vi "EVS Main Temp.vi"() -> ()   [LabVIEW 2009]
uses:
  <vilib>/vision/driver/NI_Vision_Acquisition_Software.lvlib
  <vilib>/vision/driver/IMAQdx.llb/IMAQdx Acquisition Mode.ctl
  TypeDefs/cRIO-EVS Comm/EVS to cRIO UDP packet.ctl
  UDP Lib/UDP Network Location.ctl
  <vilib>/userDefined/High Color/IMAQdx.ctl
panel:
  out "Peak":u32
  out "Processing time":u32
  in  "stop":bool
  out "Camera SICK":picture
  out "HB":bool
  in  "IMAQdx Session Left":T1="cam1" caption="Left Session"
  in  "IMAQdx Session Right":T1="cam0" caption="Right Session"
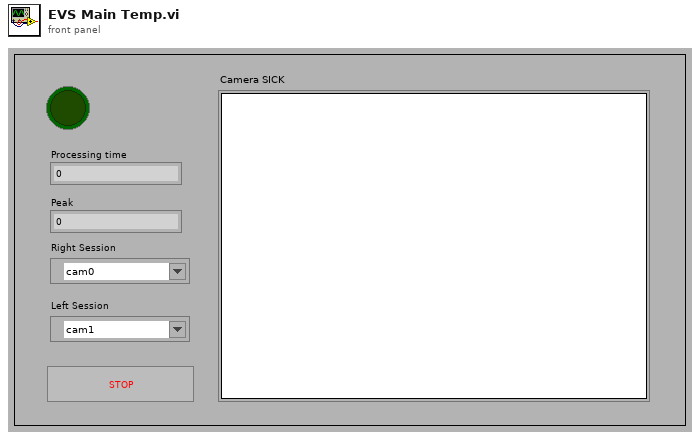
[diagram p1: front panel]
types:
  T1 = typedef "IMAQdx.ctl" = refnum<k21>
  T2 = typedef "UDP Network Location.ctl" = cluster{"IP Address":string, "Port":u16}
  T3 = typedef "EVS to cRIO UDP packet.ctl" = cluster{"Camera SICK":u16[], "Camera init":bool}
  T4 = typedef "NI_Vision_Acquisition_Software.lvlib/IMAQdx Acquisition Mode.ctl" = enum32{"One Shot", "Continuous"}
  T5 = cluster{"maximum":dbl, "minimum":dbl, "clip to min":bool, "log?(F)":bool, "grid color":u32, "plot color":u32, "fmt and prec":cluster{"format":enum8{"Decimal", "Scientific", "Engineering", "Binary", "Octal", "Hex"}, "precision":u8}, "visible section":u16}
  T6 = typedef "UDP Base.ctl" = cluster{"UDP Session":refnum<k16>, "UDP Socket Params":T7}
  T7 = typedef "UDP Socket Params.ctl" = cluster{"Local Port":u16, "Read Timeout":i32, "Write Timeout":i32}
  T8 = typedef "IMAQ Image.ctl" = refnum<image>
  T9 = cluster{"Camera SICK":u16[], ".not. x?":bool, "error out":errorcluster}
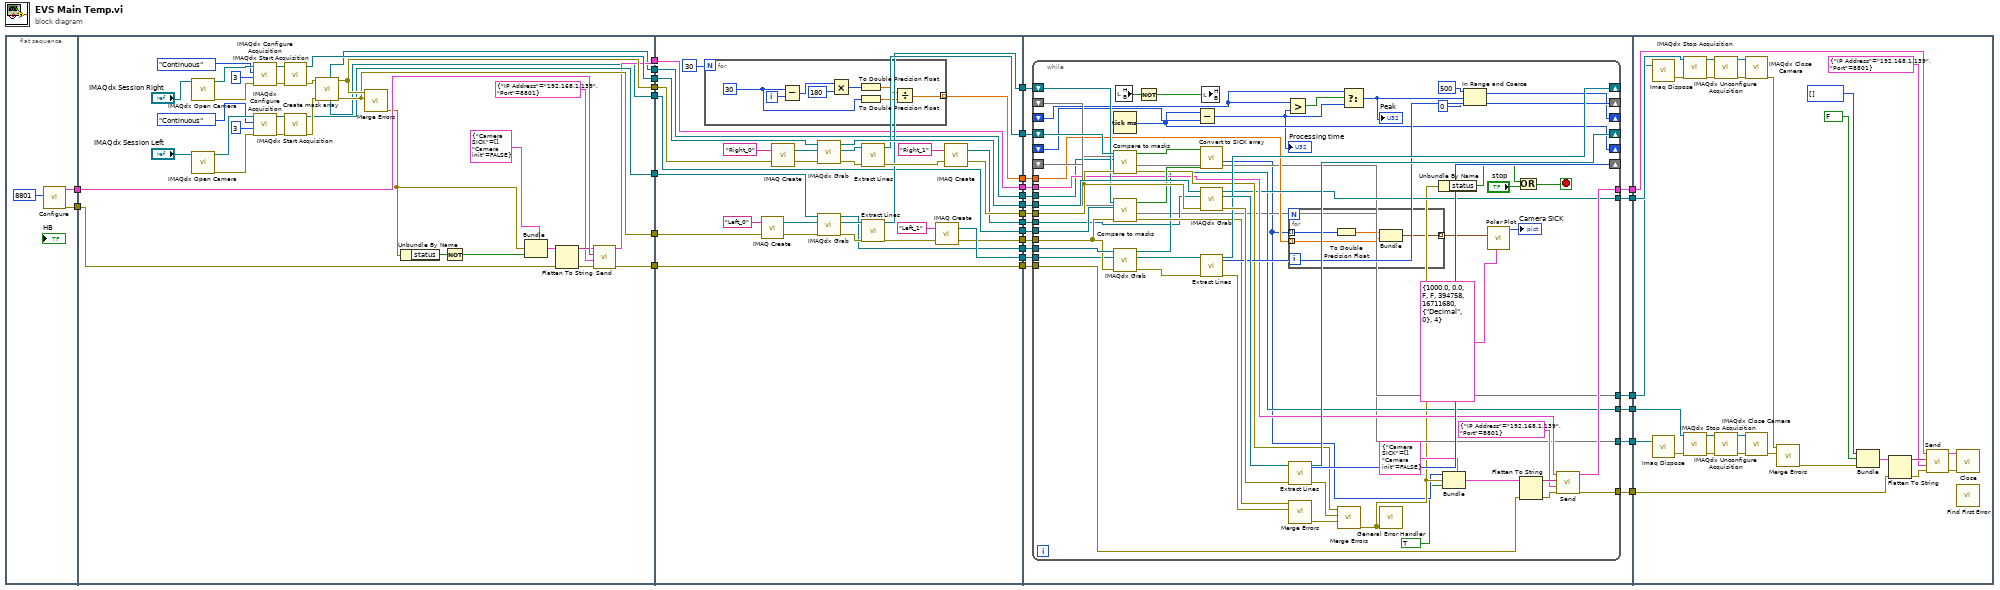
[diagram p0: block diagram]
diagram:
  n1 = flat-sequence {
    tunnel: [w31] -> w29
    tunnel: [w30] -> w28
    tunnel: w29 -> [w43]
    tunnel: w28 -> [w45]
    tunnel: [w41] -> w27
    tunnel: [w40] -> w26
    tunnel: [w39] -> w25
    tunnel: [w38] -> w24
    tunnel: [w36] -> w15
    tunnel: [w35] -> w13
    tunnel: [w34] -> w11
    tunnel: [w33] -> w10
    tunnel: w27 -> [w88]
    tunnel: w26 -> [w87]
    tunnel: w25 -> [w84]
    tunnel: w24 -> [w83]
    tunnel: [w82] -> w23
    tunnel: [w81] -> w22
    tunnel: [w78] -> w21
    tunnel: [w77] -> w20
    tunnel: [w76] -> w19
    tunnel: [w75] -> w18
    tunnel: [w74] -> w17
    tunnel: [w73] -> w16
    tunnel: w15 -> [w72]
    tunnel: [w72] -> w14
    tunnel: w13 -> [w71]
    tunnel: [w71] -> w12
    tunnel: w11 -> [w70]
    tunnel: w10 -> [w69]
    tunnel: [w70] -> w9
    tunnel: [w69] -> w8
    tunnel: [w67] -> w3
    tunnel: w23 -> [w123]
    tunnel: w22 -> [w111]
    tunnel: w21 -> [w110]
    tunnel: w20 -> [w122]
    tunnel: w19 -> [w125]
    tunnel: w18 -> [w124]
    tunnel: w17 -> [w121]
    tunnel: w16 -> [w120]
    tunnel: w14 -> [w119]
    tunnel: w12 -> [w118]
    tunnel: w9 -> [w117]
    tunnel: w8 -> [w116]
    tunnel: [w115] -> w7
    tunnel: [w114] -> w6
    tunnel: [w113] -> w5
    tunnel: [w112] -> w4
    tunnel: w3 -> [w109]
    tunnel: [w108] -> w2
    tunnel: [w107] -> w1
    tunnel: w7 -> [w209]
    tunnel: w6 -> [w208]
    tunnel: w5 -> [w200]
    tunnel: w4 -> [w199]
    tunnel: w2 -> [w194]
    tunnel: w1 -> [w192]
    frame #0 {
      n2 = call "Configure.vi"("Local Port"=u16 8801) -> ("error out"=w31:errorcluster, "UDP Base out"=w30:T6)  [unwired: 9 in]
    }
    frame #1 {
      n3 = call <vilib>:"IMAQdx Open Camera.vi"("Session In"="IMAQdx Session Right") -> ("error out"=w65:errorcluster, "Session Out"=w64:T1)  [unwired: 2 in, 7 out]
      n4 = call <vilib>:"IMAQdx Open Camera.vi"("Session In"="IMAQdx Session Left") -> ("error out"=w59:errorcluster, "Session Out"=w60:T1)  [unwired: 2 in, 7 out]
      n5 = call <vilib>:"IMAQdx Configure Acquisition.vi"("error in"=w65, "Number of Buffers"=u32 3, "Continuous?"=IMAQdx_Acquisition_Mode."Continuous", "Session In"=w64) -> ("error out"=w66:errorcluster, "Session Out"=w63:T1)  [unwired: 1 in, 5 out]
      n6 = call <vilib>:"IMAQdx Configure Acquisition.vi"("error in"=w59, "Number of Buffers"=u32 3, "Continuous?"=IMAQdx_Acquisition_Mode."Continuous", "Session In"=w60) -> ("error out"=w58:errorcluster, "Session Out"=w61:T1)  [unwired: 1 in, 5 out]
      n7 = call <vilib>:"IMAQdx Start Acquisition.vi"("error in"=w66, "Session In"=w63) -> ("error out"=w52:errorcluster, "Session Out"=w38:T1)  [unwired: 8 out]
      n8 = call <vilib>:"IMAQdx Start Acquisition.vi"("error in"=w58, "Session In"=w61) -> ("error out"=w51:errorcluster, "Session Out"=w39:T1)  [unwired: 8 out]
      n9 = call "Create mask array.vi"("Left error in"=w51, "Right Error in"=w52) -> ("Left error out"=w40:errorcluster, "Right error out"=w41:errorcluster, "Left Cam Masks"=w33:T8[], "Right Cam Masks"=w34:T8[])  [unwired: 6 in]
      n10 = call <vilib>:"Merge Errors.vi"("error in 2 (no error)"=w40, "error in 1 (no error)"=w41) -> ("error out"=w37:errorcluster)  [unwired: 5 in]
      n11 = Unbundle By Name(w37) -> ("status"=w50:bool)
      n12 = Not(x=w50) -> (.not. x?=w46:bool)
      n13 = Bundle(cluster=T3 {"Camera SICK"=[], "Camera init"=FALSE} ("EVS to cRIO UDP packet"), w37, w46) -> (w49:T3)  [unwired: 1 in]
      n14 = Flatten To String(anything=w49, error in (no error)=w43) -> (data string=w48:string, error out=w42:errorcluster)  [unwired: 2 in, 1 out]
      n15 = call "Send.vi"("error in (no error)"=w42, "Destination Location"=T2 {"IP Address"="192.168.1.139", "Port"=8801}, "Send Data"=w48, "UDP Base in"=w45) -> ("error out"=w35:errorcluster, "UDP Base out"=w36:T6)  [unwired: 5 in, 1 out]
    }
    frame #2 {
      n16 = for {
        N: 30 -> [_]
        tunnel: [w102] -> w67 mode=indexing
        i -> [w106]
        w104 = 30 ("x")
        n17 = Subtract(x=w104, y=w106) -> (x-y=w103:i32)
        n18 = Multiply(x=w103, y=180) -> (x*y=w101:i32)
        n19 = To Double Precision Float(number=w101) -> (double precision float=w99:dbl)
        n20 = To Double Precision Float(number=w104) -> (double precision float=w100:dbl)
        n21 = Divide(x=w99, y=w100) -> (x/y=w102:dbl)
      }
      n22 = call "IMAQ Create"("Image Name"="Left_0", "error in (no error)"=w87) -> ("New Image"=w92:T8, "error out"=w91:errorcluster)  [unwired: 3 in]
      n23 = call "IMAQ Create"("Image Name"="Right_0", "error in (no error)"=w88) -> ("New Image"=w90:T8, "error out"=w89:errorcluster)  [unwired: 3 in]
      n24 = call <vilib>:"IMAQdx Grab.vi"("error in"=w89, "Image In"=w90, "Session In"=w83) -> ("error out"=w97:errorcluster, "Image Out"=w93:T8, "Session Out"=w76:T1)  [unwired: 5 in, 1 out]
      n25 = call <vilib>:"IMAQdx Grab.vi"("error in"=w91, "Image In"=w92, "Session In"=w84) -> ("error out"=w96:errorcluster, "Image Out"=w94:T8, "Session Out"=w75:T1)  [unwired: 5 in, 1 out]
      n26 = call "Extract Lines.vi"("error in (no error)"=w97, "Image Src"=w93) -> ("error out"=w98:errorcluster, "Image Out"=w74:T8)  [unwired: 7 in, 1 out]
      n27 = call "Extract Lines.vi"("error in (no error)"=w96, "Image Src"=w94) -> ("error out"=w95:errorcluster, "Image Out"=w73:T8)  [unwired: 7 in, 1 out]
      n28 = call "IMAQ Create"("Image Name"="Left_1", "error in (no error)"=w95) -> ("New Image"=w78:T8, "error out"=w77:errorcluster)  [unwired: 3 in]
      n29 = call "IMAQ Create"("Image Name"="Right_1", "error in (no error)"=w98) -> ("New Image"=w81:T8, "error out"=w82:errorcluster)  [unwired: 3 in]
    }
    frame #3 {
      n30 = while {
        tunnel: w125 -> [w182]
        tunnel: w124 -> [w181]
        tunnel: w123 -> [w179]
        tunnel: w122 -> [w180]
        shift-right: [w177] -> _
        shift-left: w121 -> [w178]
        shift-right: [w175] -> _
        shift-left: w120 -> [w176]
        shift-right: [w172] -> _
        shift-left: _ -> [w171]
        shift-right: [w170] -> _
        shift-left: _ -> [w169]
        tunnel: w119 -> [w162]
        tunnel: w118 -> [w161]
        tunnel: [w158] -> w113
        tunnel: [w157] -> w112
        tunnel: w117 -> [w156]
        tunnel: w116 -> [w155]
        tunnel: [w154] -> w114
        tunnel: [w153] -> w115
        tunnel: w111 -> [w152]
        tunnel: w110 -> [w151]
        tunnel: w109 -> [w148]
        shift-right: [w142] -> _
        shift-left: _ -> [w143]
        tunnel: [w139] -> w108
        tunnel: [w138] -> w107
        shift-right: [w134] -> _
        shift-left: _ -> [w135]
        stop <- w146 stop-if-true
        n31 = Tick Count (ms)() -> (millisecond timer value=w142:u32)
        n32 = call "Compare to masks.vi"("Number of Particles1"=w169, "error in (no error)"=w179, "Mask array"=w156, "Image Src"=w178) -> ("Final error out"=w167:errorcluster, 1:w139, "Marked Regions"=w174:bool[])  [unwired: 5 in]
        n33 = call "Compare to masks.vi"("Number of Particles1"=w171, "error in (no error)"=w180, "Mask array"=w155, "Image Src"=w176) -> ("Final error out"=w165:errorcluster, 1:w138, "Marked Regions"=w173:bool[])  [unwired: 5 in]
        n34 = call <vilib>:"IMAQdx Grab.vi"("error in"=w180, "Image In"=w151, "Session In"=w181) -> ("error out"=w183:errorcluster, "Image Out"=w184:T8, "Session Out"=w153:T1)  [unwired: 5 in, 1 out]
        n35 = local read "HB"() -> (w150:bool)
        n36 = Not(x=w150) -> (.not. x?=w149:bool)
        n37 = Subtract(x=w142, y=w143) -> (x-y=w136:u32)
        "Processing time" <- w136
        n38 = call "Convert to SICK array.vi"("Left Regions"=w173, "Right Regions"=w174) -> ("Sick array"=w128:u16[])  [unwired: 9 in]
        n39 = call <vilib>:"IMAQdx Grab.vi"("error in"=w179, "Image In"=w152, "Session In"=w182) -> ("error out"=w185:errorcluster, "Image Out"=w186:T8, "Session Out"=w154:T1)  [unwired: 5 in, 1 out]
        n40 = call "Extract Lines.vi"("error in (no error)"=w183, "Image Src"=w184) -> ("error out"=w164:errorcluster, "Image Out"=w175:T8, "Extraction mode"=w172:i32)  [unwired: 6 in, 1 out]
        n41 = local write "HB"(w149) -> ()
        n42 = Greater?(x=w135, y=w136) -> (0:w137:bool)
        n43 = for {
          tunnel: w128 -> [w190] mode=indexing
          tunnel: [w189] -> w140 mode=indexing
          tunnel: w148 -> [w188] mode=indexing
          n44 = To Double Precision Float(number=w190) -> (double precision float=w187:dbl)
          n45 = Bundle(w187, w188) -> (w189:cluster{dbl, dbl})  [unwired: 1 out]
        }
        n46 = call "Extract Lines.vi"("error in (no error)"=w185, "Image Src"=w186) -> ("error out"=w166:errorcluster, "Image Out"=w177:T8, "Extraction mode"=w170:i32)  [unwired: 6 in, 1 out]
        n47 = call <vilib>:"Merge Errors.vi"("error in 2 (no error)"=w164, "error in 1 (no error)"=w165) -> ("error out"=w163:errorcluster)  [unwired: 5 in]
        n48 = call <vilib>:"Merge Errors.vi"("error in 3 (no error)"=w163, "error in 2 (no error)"=w166, "error in 1 (no error)"=w167) -> ("error out"=w129:errorcluster)  [unwired: 4 in]
        n49 = Select(t=w135, s=w137, f=w136) -> (s? t:f=w133:u32)
        "Peak" <- w133
        n50 = call <vilib>:"General Error Handler.vi"("error in (no error)"=w129) -> ()  [unwired: 10 in, 5 out]
        n51 = Unbundle By Name(w129) -> ("status"=w145:bool)
        n52 = Bundle(cluster=T3 {"Camera SICK"=[], "Camera init"=FALSE} ("EVS to cRIO UDP packet"), w128, w129, TRUE (".not. x?")) -> (w126:T3)
        n53 = In Range and Coerce(upper limit=u32 500, x=w133, lower limit=u32 0) -> (coerced(x)=w134:u32)  [unwired: 1 out]
        n54 = call <vilib>:"Polar Plot.vi"("polar attributes"=T5 {"maximum"=1000.0, "minimum"=0.0, "clip to min"=FALSE, "log?(F)"=FALSE, "grid color"=394758, "plot color"=16711680, "fmt and prec"={"format"=enum."Decimal", "precision"=0}, "visible section"=4}, "data array [mag, phase (deg)]"=w140) -> ("new picture"=→"Camera SICK":picture)  [unwired: 1 in, 8 out]
        n55 = Or(x=w145, y="stop") -> (x .or. y?=w146:bool)
        n56 = Flatten To String(anything=w126, error in (no error)=w161) -> (data string=w168:string, error out=w160:errorcluster)  [unwired: 2 in, 1 out]
        n57 = call "Send.vi"("error in (no error)"=w160, "Destination Location"=T2 {"IP Address"="192.168.1.139", "Port"=8801}, "Send Data"=w168, "UDP Base in"=w162) -> ("error out"=w157:errorcluster, "UDP Base out"=w158:T6)  [unwired: 5 in, 1 out]
      }
    }
    frame #4 {
      n58 = call "Imaq Dispose"("Image"=w194) -> ("error out"=w193:errorcluster)  [unwired: 5 in]
      n59 = call "Imaq Dispose"("Image"=w192) -> ("error out"=w191:errorcluster)  [unwired: 5 in]
      n60 = call <vilib>:"IMAQdx Stop Acquisition.vi"("error in"=w193, "Session In"=w208) -> ("error out"=w215:errorcluster, "Session Out"=w214:T1)  [unwired: 8 out]
      n61 = call <vilib>:"IMAQdx Stop Acquisition.vi"("error in"=w191, "Session In"=w209) -> ("error out"=w211:errorcluster, "Session Out"=w210:T1)  [unwired: 8 out]
      n62 = call <vilib>:"IMAQdx Unconfigure Acquisition.vi"("error in"=w215, "Session In"=w214) -> ("error out"=w216:errorcluster, "Session Out"=w217:T1)  [unwired: 8 out]
      n63 = call <vilib>:"IMAQdx Unconfigure Acquisition.vi"("error in"=w211, "Session In"=w210) -> ("error out"=w212:errorcluster, "Session Out"=w213:T1)  [unwired: 8 out]
      n64 = call <vilib>:"IMAQdx Close Camera.vi"("error in"=w216, "Session In"=w217) -> ("error out"=w207:errorcluster)  [unwired: 9 out]
      n65 = call <vilib>:"IMAQdx Close Camera.vi"("error in"=w212, "Session In"=w213) -> ("error out"=w206:errorcluster)  [unwired: 9 out]
      n66 = call <vilib>:"Merge Errors.vi"("error in 2 (no error)"=w206, "error in 1 (no error)"=w207) -> ("error out"=w198:errorcluster)  [unwired: 5 in]
      n67 = Bundle("Camera SICK"=u16[] [], ".not. x?"=FALSE, "error out"=w198) -> (w204:T9)  [unwired: 1 in]
      n68 = Flatten To String(anything=w204, error in (no error)=w199) -> (data string=w205:string, error out=w202:errorcluster)  [unwired: 2 in, 1 out]
      n69 = call "Send.vi"("error in (no error)"=w202, "Destination Location"=T2 {"IP Address"="192.168.1.139", "Port"=8801}, "Send Data"=w205, "UDP Base in"=w200) -> ("error out"=w195:errorcluster, "UDP Base out"=w196:T6)  [unwired: 5 in, 1 out]
      n70 = call "Close.vi"("error in (no error)"=w195, "Cluster of class private data"=w196) -> ()  [unwired: 9 in, 1 out]
      n71 = call <vilib>:"Find First Error.vi"() -> ()  [unwired: 4 in, 2 out]
    }
  }
